vi "TwGetTimingDataLV.vi"(0 "error in (no error)":errorcluster, 1 "filename":string, 10 "bufOffset":i32, 11 "bufCount":i32, 12 "writeOffset":i32, 13 "writeCount":i32) -> (14 "error out":errorcluster, 19 "dataBuffer":dbl[](array[numeric]))   [LabVIEW 2009]
uses:
  TwH5Dll.dll
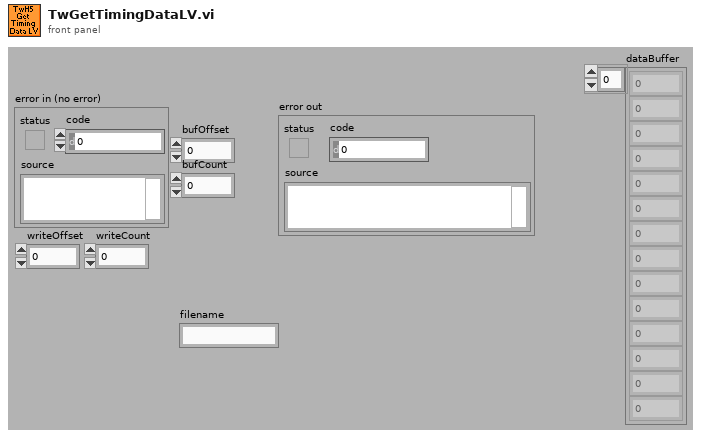
[diagram p1: front panel]
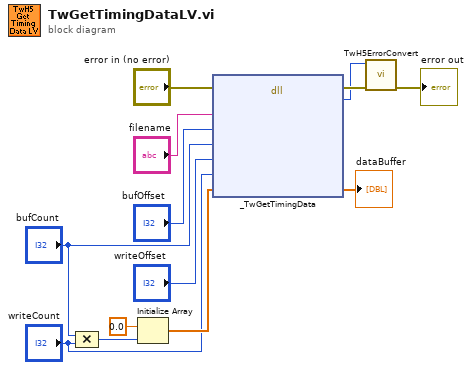
[diagram p0: block diagram]
diagram:
  n1 = Compound Arithmetic op=MULTIPLY("bufCount", "writeCount") -> (w1:i32)
  n2 = Initialize Array(0.0 ("element"), w1) -> (w5:dbl[])
  n3 = dll-call lib="C:/src/85_TofDaq_current/DllWrappers/LabView/TwH5Dll/TwH5Dll.dll" fn="_TwGetTimingData"(error in="error in (no error)", "filename"="filename", "bufOffset"="bufOffset", "bufCount"="bufCount", "writeOffset"="writeOffset", "writeCount"="writeCount", "dataBuffer"=w5) -> (error out=w12:errorcluster, "TwRetVal"=w11:i32, "dataBuffer"=→"dataBuffer":dbl[])  [unwired: 7 in, 1 out]
  n4 = call "TwH5ErrorConvert.vi"("error in (no error)"=w12, "error code"=w11) -> ("error out"=→"error out":errorcluster)  [unwired: 9 out]
